vi "Start.vi"(8 "error in (no error)":errorcluster, 10 "Message in":refnum<class "StartMessage.lvclass">, 11 "ImageStack in":refnum<class "ImageStack.lvclass">) -> (0 "error out":errorcluster, 3 "ImageStack out":refnum<class "ImageStack.lvclass">)   [LabVIEW 2012, in "ImageStack.lvclass"]
doc: "This member function is called when the statemachine in the run.vi receives an 'start' command. It relays the message to all observers of the component.\n\nOverride this member function in your derived class if you need additional start functionality (but don't forget to call the parent method)."
uses:
  ImageStack.lvclass
  <vilib>/Distrio/Murmex/StartMessage/StartMessage.lvclass
  <vilib>/Distrio/Murmex/StartMessage/run mode enum.ctl
  ImageStack.lvclass/ImageStack.ctl
  <vilib>/Distrio/Murmex/Murmex/Murmex.lvclass
panel:
  # "This member function is called when the statemachine in the run.vi receives an 'start' command. It relays the message to all observers of the component.\n\nOverride this member function in your derived class if you need additional start functionality (but don't forget to call the parent method)."
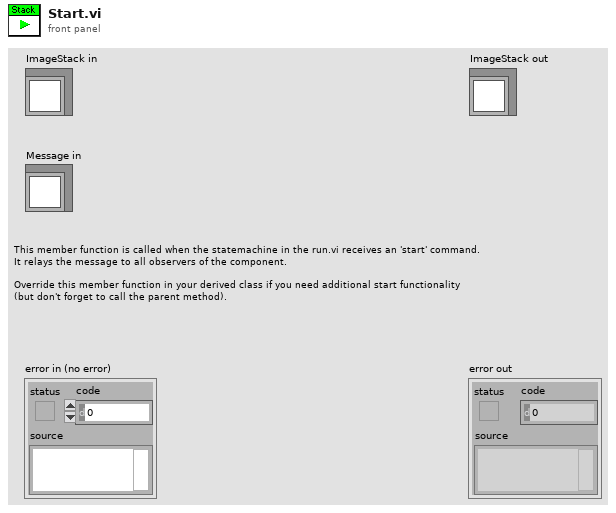
[diagram p1: front panel]
types:
  T1 = typedef "Murmex.lvlib/StartMessage.lvclass/run mode enum.ctl" = enum16{"infinite", "finite"}
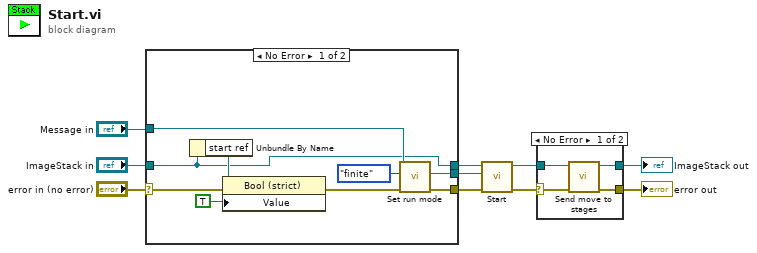
[diagram p0: block diagram]
diagram:
  n1 = case shown="No Error" "error in (no error)" {
    selector: "error in (no error)" -> [w14 w22]
    tunnel: [w18 w22] -> w7
    tunnel: [w12 w21] -> w9
    tunnel: "Message in" -> [w19 w20]
    tunnel: [w16 w20] -> w8
    tunnel: "ImageStack in" -> [w12 w21]
    frame No Error {
      n2 = Unbundle By Name(w12) -> ("start ref"=w15:refnum<vi>)
      n3 = property class="Bool (strict)"(reference=w15, error in=w14, "Value"=TRUE) -> (error out=w11:errorcluster)  [unwired: 1 out]
      n4 = call <vilib>:"Set run mode.vi"("error in (no error)"=w11, "run mode"=run_mode_enum."finite", "StartMessage in"=w19) -> ("error out"=w18:errorcluster, "StartMessage out"=w16:refnum<class "StartMessage.lvclass">)  [unwired: 7 in]
    }
    frame Error {
    }
  }
  n5 = call-parent "Start.vi"("error in (no error)"=w7, "Message in"=w8, "Murmex in"=w9) -> ("error out"=w4:errorcluster, "Murmex out"=w2:refnum<class "ImageStack.lvclass">)  [unwired: 7 in]
  n6 = case shown="No Error" w4 {
    selector: w4 -> [w26 w27]
    tunnel: [w25 w27] -> w3
    tunnel: w2 -> [w24 w28]
    tunnel: [w23 w28] -> w1
    frame No Error {
      n7 = call-dynamic "Send move to stages.vi"("error in (no error)"=w26, "ImageStack in"=w24) -> ("error out"=w25:errorcluster, "ImageStack out"=w23:refnum<class "ImageStack.lvclass">)  [unwired: 8 in]
    }
    frame Error {
    }
  }
  "error out" <- w3
  "ImageStack out" <- w1
